vi "Show Animated Busy Icon with Message and Abort Button.vi"(2 "Already active? (F)":bool, 3 "Message":string, 7 "Target VI reference":refnum<vi>, 11 "Error In":errorcluster, 16 "Abort Button Name (Abort)":string="Abort", 17 "Animated Busy Icon Control Name (Animated Busy Icon)":string="Animated Busy Icon", 18 "Message Control Name (Message)":string="Message") -> (10 "Error Out":errorcluster)   [LabVIEW 2019]
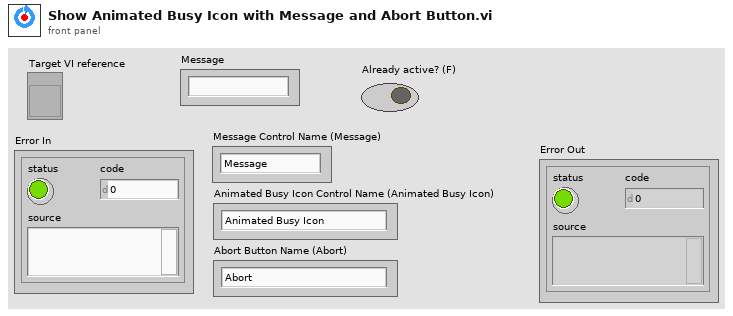
[diagram p1: front panel]
types:
  T1 = enum16{"Controls & Indicators", "Controls", "Indicators"}
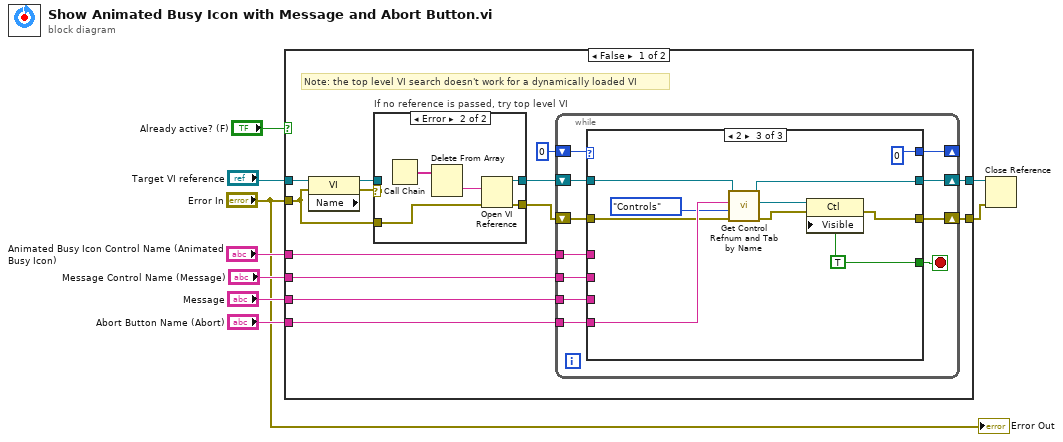
[diagram p0: block diagram]
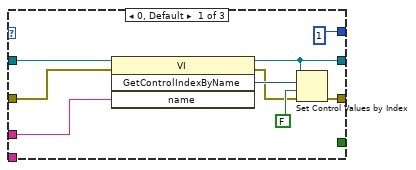
[diagram p3: hidden frame]
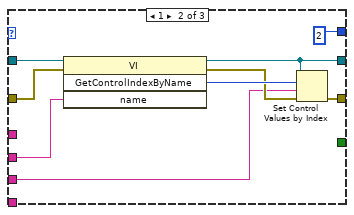
[diagram p4: hidden frame]
diagram:
  n1 = case shown="False" "Already active? (F)" {
    tunnel: [w20 w69] -> w9
    tunnel: [w19 _] -> w8
    tunnel: "Message Control Name (Message)" -> [w17 _]
    tunnel: "Animated Busy Icon Control Name (Animated Busy Icon)" -> [w16 _]
    tunnel: "Message" -> [w15 _]
    tunnel: "Target VI reference" -> [w14 w69]
    tunnel: "Error In" -> [w10 _]
    tunnel: "Abort Button Name (Abort)" -> [w11 _]
    frame False {
      # "Note: the top level VI search doesn't work for a dynamically loaded VI"
      n2 = property class="VI" props=["Name"](reference=w14, error in=w10) -> (reference out=w12:refnum<vi>, error out=w13:errorcluster)  [unwired: 1 out]
      n3 = case "If no reference is passed, try top level VI" shown="Error" w13 {
        selector: w13 -> [w23 _]
        tunnel: [w23 w29] -> w22
        tunnel: [w24 w28] -> w21
        tunnel: w12 -> [w24 _]
        tunnel: w10 -> [_ w25]
        frame No Error {
        }
        frame Error {
          n4 = Call Chain() -> (call chain=w26:string[])
          n5 = Delete From Array(array=w26) -> (deleted portion=w27:string)  [unwired: 2 in, 1 out]
          n6 = Open VI Reference(vi path=w27, error in (no error)=w25) -> (vi reference=w28:refnum<vi>, error out=w29:errorcluster)  [unwired: 4 in]
        }
      }
      n7 = while {
        shift-right: [w37] -> w19
        shift-left: w22 -> [w40]
        shift-right: [w38] -> w20
        shift-left: w21 -> [w39]
        shift-right: [w35] -> _
        shift-left: 0 -> [w36]
        tunnel: w17 -> [w33]
        tunnel: w16 -> [w32]
        tunnel: w15 -> [w31]
        tunnel: w11 -> [w30]
        stop <- w34 stop-if-true
        n8 = case shown="2" w36 {
          tunnel: w40 -> [w46 w56 w66]
          tunnel: w39 -> [w45 w55 w64]
          tunnel: [w44 w54 w63] -> w38
          tunnel: [w43 w53 w60] -> w37
          tunnel: [1 2 0] -> w35
          tunnel: [_ _ w59] -> w34
          tunnel: w33 -> [_ w51 _]
          tunnel: w32 -> [w41 _ _]
          tunnel: w31 -> [_ w50 _]
          tunnel: w30 -> [_ _ w67]
          frame 0, Default {
            n9 = invoke class="VI" method="GetControlIndexByName"(reference=w45, error in=w46, "name"=w41) -> (reference out=w44:refnum<vi>, error out=w47:errorcluster, "GetControlIndexByName"=w49:i32)  [unwired: 1 in, 1 out]
            n10 = Set Control Values by Index(0:w44, 1:w49, 2:FALSE ("Visible"), 3:w47) -> (11:w43:errorcluster)
          }
          frame 1 {
            n11 = invoke class="VI" method="GetControlIndexByName"(reference=w55, error in=w56, "name"=w51) -> (reference out=w54:refnum<vi>, error out=w57:errorcluster, "GetControlIndexByName"=w58:i32)  [unwired: 1 in, 1 out]
            n12 = Set Control Values by Index(0:w54, 1:w58, 2:w50, 3:w57) -> (11:w53:errorcluster)
          }
          frame 2 {
            w59 = TRUE
            n13 = call "Get Control Refnum and Tab by Name.vi"("error in"=w66, "Selection"=T1."Controls", "Control Label"=w67, "VI  Ref"=w64) -> ("error out"=w61:errorcluster, "Ctl Refnum"=w62:refnum<vi>, "VI  Ref (out)"=w63:refnum<vi>)  [unwired: 3 in, 2 out]
            n14 = property class="Ctl"(reference=w62, error in=w61, "Visible"=w59) -> (error out=w60:errorcluster)  [unwired: 1 out]
          }
        }
      }
    }
    frame True {
    }
  }
  n15 = Close Reference(reference=w9, error in (no error)=w8) -> ()  [unwired: 1 out]
  "Error Out" <- "Error In"
